vi "Configure Modulation.vi"   [LabVIEW 2020, in "Template - Function Generator.lvlib"]
doc: "Allows users to configure different modulation settings on the function generator."
uses:
  <instrlib>/_Template - Function Generator/Template - Function Generator.lvlib
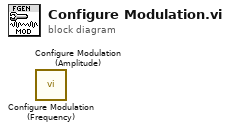
[diagram p0: block diagram]
diagram:
  n1 = call <instrlib>:"Configure Modulation (Frequency).vi"() -> ()  [unwired: 10 in, 2 out]
  n2 = call <instrlib>:"Configure Modulation (Amplitude).vi"() -> ()  [unwired: 10 in, 2 out]
